vi "turbine.vi"() -> ()   [LabVIEW 2018]
panel:
  out "Speed Guage -\nBlades Failure for Speeds Above 350":dbl(knob) scale=0.0..420.0
  in  "Table Control":string[][](table)
  out "Power Meter":dbl(knob) scale=0.0..400000.0
  out "Y_Axis Speed":dbl(graph)
  out "X_Axis Speed":dbl(graph)
  out "Blades":bool
  out "Ring":u16(ring)
  in  "Wind Speed":dbl[](array[slide]) scale=0.0..420.0
  out "Turbine Height for Optimal Power generation":i32[](array[numeric])
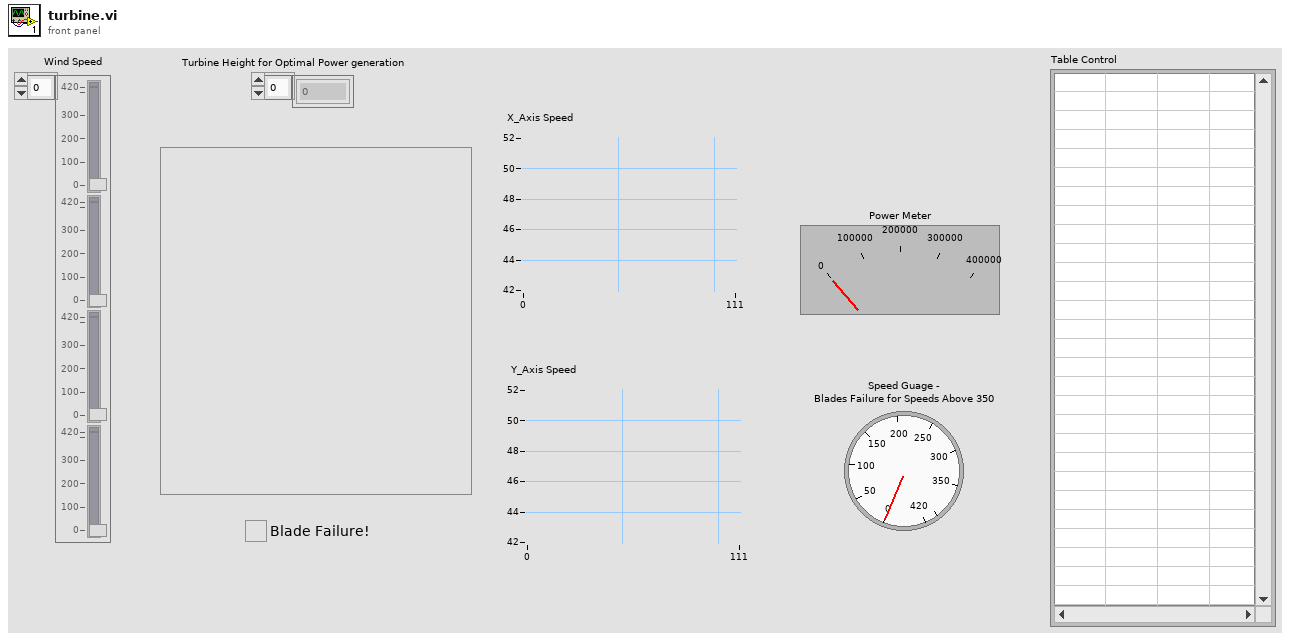
[diagram p1: front panel]
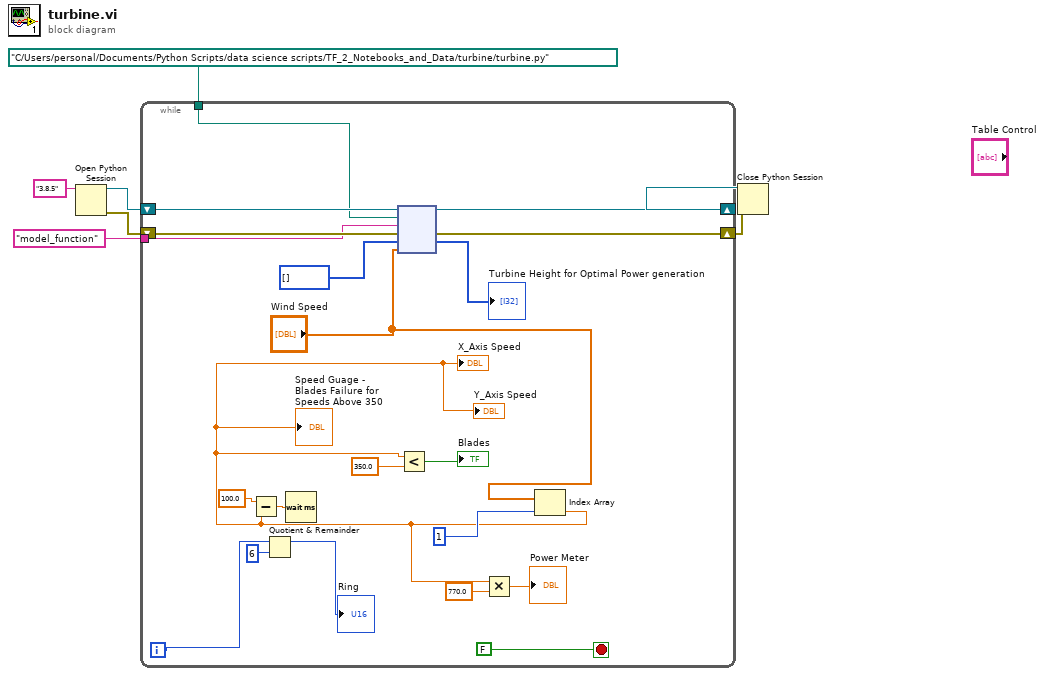
[diagram p0: block diagram]
diagram:
  n1 = Open Python Session(python version="3.8.5" ("Python version")) -> (session out=w7:refnum<k35>, error out=w6:errorcluster)  [unwired: 2 in]
  n2 = while {
    tunnel: path "C:/Users/personal/Documents/Python Scripts/data science scripts/TF_2_Notebooks_and_Data/turbine/turbine.py" ("module path") -> [w24]
    tunnel: "model_function" ("function name") -> [w23]
    shift-right: [w26] -> w5
    shift-left: w7 -> [w28]
    shift-right: [w25] -> w4
    shift-left: w6 -> [w27]
    i -> [w13]
    stop <- FALSE stop-if-true
    n3 = Quotient & Remainder(x=w13, y=6) -> (x-y*floor(x/y)=→"Ring":i32)  [unwired: 1 out]
    n4 = node(w28, w24, w23, w27, i32[] [], "Wind Speed") -> (w26:refnum<k35>, w25:errorcluster, →"Turbine Height for Optimal Power generation":i32[])  [unwired: 1 in, 2 out]
    n5 = Index Array(array="Wind Speed", index=1) -> (element=w8:dbl)
    "X_Axis Speed" <- w8
    "Y_Axis Speed" <- w8
    "Speed Guage -\nBlades Failure for Speeds Above 350" <- w8
    n6 = Subtract(x=100.0, y=w8) -> (x-y=w14:dbl)
    n7 = Wait (ms)(milliseconds to wait=w14) -> ()  [unwired: 1 out]
    n8 = Less?(x=w8, y=350.0) -> (x < y?=→"Blades":bool)
    n9 = Multiply(x=w8, y=770.0) -> (x*y=→"Power Meter":dbl)
  }
  n10 = Close Python Session(session in=w5, error in=w4) -> ()  [unwired: 1 out]
